vi "IPI_Cal_Laser_X_Pos.vi"(10 "X Distance":string, 11 "X pos":dbl[](array[numeric])) -> (3 "X Laser Pos":dbl[](array[numeric]))   [LabVIEW 2015]
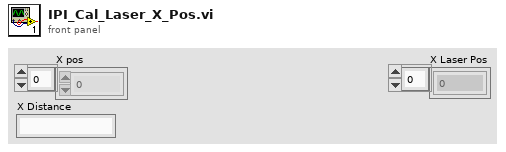
[diagram p1: front panel]
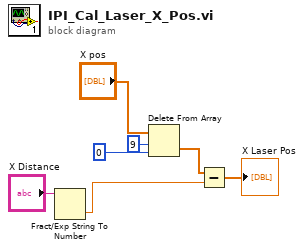
[diagram p0: block diagram]
diagram:
  n1 = Fract/Exp String To Number(string="X Distance") -> (number=w2:dbl)  [unwired: 3 in, 1 out]
  n2 = Delete From Array(array="X pos", length=9 ("长度"), index=0 ("索引")) -> (deleted portion=w3:dbl[])  [unwired: 1 out]
  n3 = Subtract(x=w3, y=w2) -> (x-y=→"X Laser Pos":dbl[])
